vi "ARydh_get_voltage -- V1.vi"(4 "Oscillator (0)":u16, 8 "Error In":errorcluster, 9 "timeconstant (s)":dbl=0.006, 10 "Freq IN (Hz)":dbl=40000.0 format="%#_13g", 11 "MCL object":T1) -> (0 "Error Out":errorcluster, 1 "z out (V)":cdb, 2 "Freq out (Hz)":dbl=40000.0 format="%#_13g", 3 "MCL object OUT":T1)   [LabVIEW 2018]
uses:
  Users/Nanocal/Desktop/Calorimetry v1.3/MCL.lvlibp/MCL library/MCL_DataRef.ctl
  Users/Nanocal/Desktop/Calorimetry v1.3/MCL.lvlibp/SynkTek FPGA/FPGA_SharedResources/FPGASharedResources_Lockin_Typedef.ctl
  Arydh  lockin fields.ctl
  Users/Nanocal/Desktop/Calorimetry v1.3/MCL.lvlibp
  Users/Nanocal/Desktop/Calorimetry v1.3/MCL.lvlibp/SynkTek FPGA/FPGA_SharedResources/FPGA_SharedResources.lvlib
panel:
  out "Phase OUT (deg)":dbl=40000.0 format="%#_13g"
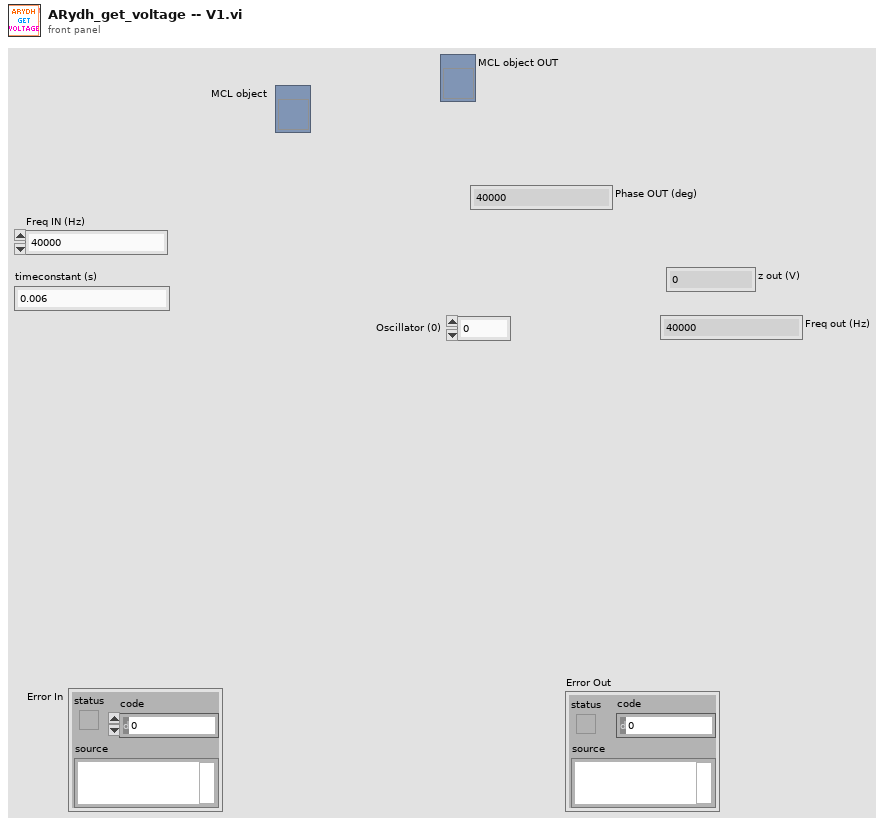
[diagram p1: front panel]
types:
  T1 = typedef "MCL.lvlibp/MCL_DataRef.ctl" = refnum<vi>
  T2 = typedef "Arydh  lockin fields.ctl" = enum16{"AV1", "AV2", "BV1", "BV2", "CV1", "CV2", "DV1", "DV2", "EV1", "EV2", "AI", "BI", "CI", "DI", "EI", "int"}
  T3 = typedef "MCL.lvlibp/FPGA_SharedResources.lvlib/FPGASharedResources_Lockin_Typedef.ctl" = enum8{"Lock-in set L1", "Lock-in set L2"}
  T4 = typedef "MCL.lvlibp/LIData.lvlib/LIData_DataReadings_typedef.ctl" = cluster{"DC":dbl[], "X":dbl[], "Y":dbl[], "R":dbl[], "theta (deg)":dbl[]}
  T5 = typedef "MCL.lvlibp/LIData.lvlib/LIData_Readings_Typedef.ctl" = cluster{"dt (s)":dbl, "Cycles per sample":dbl, "Sync index":dbl, "Point number":dbl, "Lock-in f (Hz)":dbl, "Module data":cluster{"Digital in f (Hz)":dbl, "Digital out f (Hz)":dbl, "Amplitude (Vrms)":dbl, "Output offset (V)":dbl}[], "PLL 1 (Hz)":dbl, "PLL 2 (Hz)":dbl, "Composite 1 (Hz)":dbl}
  T6 = cluster{"Digital in f (Hz)":dbl, "Digital out f (Hz)":dbl, "Amplitude (Vrms)":dbl, "Output offset (V)":dbl}[]
  T7 = cluster{"Digital in f (Hz)":dbl, "Digital out f (Hz)":dbl, "Amplitude (Vrms)":dbl, "Output offset (V)":dbl}
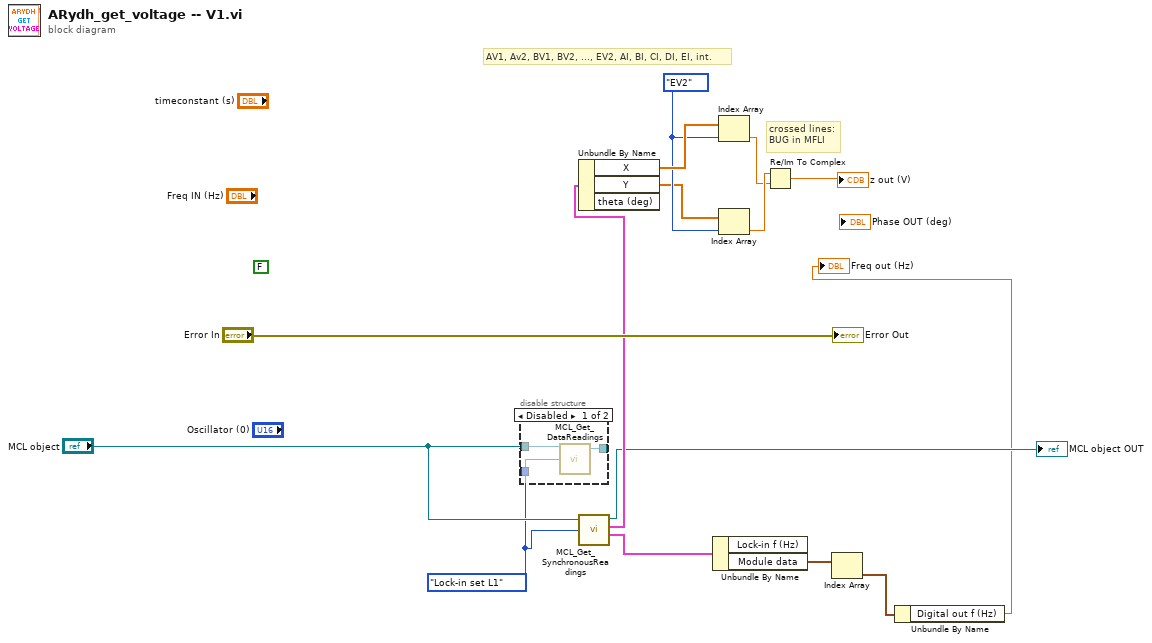
[diagram p0: block diagram]
diagram:
  w13 = Arydh__lockin_fields."EV2"
  w2 = FPGASharedResources_Lockin_Typedef."Lock-in set L1" ("Lockin")
  (unwired) FALSE
  # "AV1, Av2, BV1, BV2, ..., EV2, AI, BI, CI, DI, EI, int."
  # "crossed lines:\nBUG in MFLI"
  n1 = disable-structure shown="Disabled" {
    disable-tunnel: "MCL object" -> [w18 _]
    disable-tunnel: [w17 _] -> _
    disable-tunnel: w2 -> [w16 _]
    frame Disabled {
      n2 = call "MCL_Get_DataReadings.vi"("Lockin"=w16, "MCL object"=w18) -> ("MCL object"=w17:T1)  [unwired: 1 in, 2 out]
    }
    frame Enabled {
    }
  }
  n3 = call "MCL_Get_SynchronousReadings.vi"("MCL object"="MCL object", "Lockin"=w2) -> ("MCL object"=→"MCL object OUT":T1, "DataReadings"=w8:T4, "GeneralReadings"=w7:T5)  [unwired: 1 in, 1 out]
  n4 = Unbundle By Name(w8) -> ("X"=w14:dbl[], "Y"=w12:dbl[])  [unwired: 1 out]
  n5 = Unbundle By Name(w7) -> ("Module data"=w6:T6)  [unwired: 1 out]
  n6 = Index Array(array=w14, index=w13) -> (element=w10:dbl)
  n7 = Index Array(array=w12, index=w13) -> (element=w11:dbl)
  n8 = Re/Im To Complex(1:w10, 2:w11) -> (0:→"z out (V)":cdb)
  n9 = Index Array(array=w6) -> (element=w5:T7)  [unwired: 1 in]
  n10 = Unbundle By Name(w5) -> ("Digital out f (Hz)"=→"Freq out (Hz)":dbl)
  "Error Out" <- "Error In"
